vi "Main.vi"() -> ()   [LabVIEW 2014, in "LinksApplication.lvclass"]
uses:
  LinksApplication.lvclass
  Featherweight/Core/Actor/Instance/FTW-Actor.lvclass
  Featherweight/Core/Actor/Reference/FTW-ActorReference.lvclass
  Featherweight/Web/Server/FTW-WebService.lvclass
  <vilib>/wsapi/Web Request.lvclass
  Featherweight/Web/Utils/FTW-Web-HTTPResponseCode.ctl
  System.Windows.Forms
panel:
  in  "Canvas":refnum<k24>(container)
types:
  T1 = typedef "FTW-Web-HTTPResponseCode.ctl" = i32
  T2 = cluster{"Incoming HTTP Request":refnum<event-registration>}
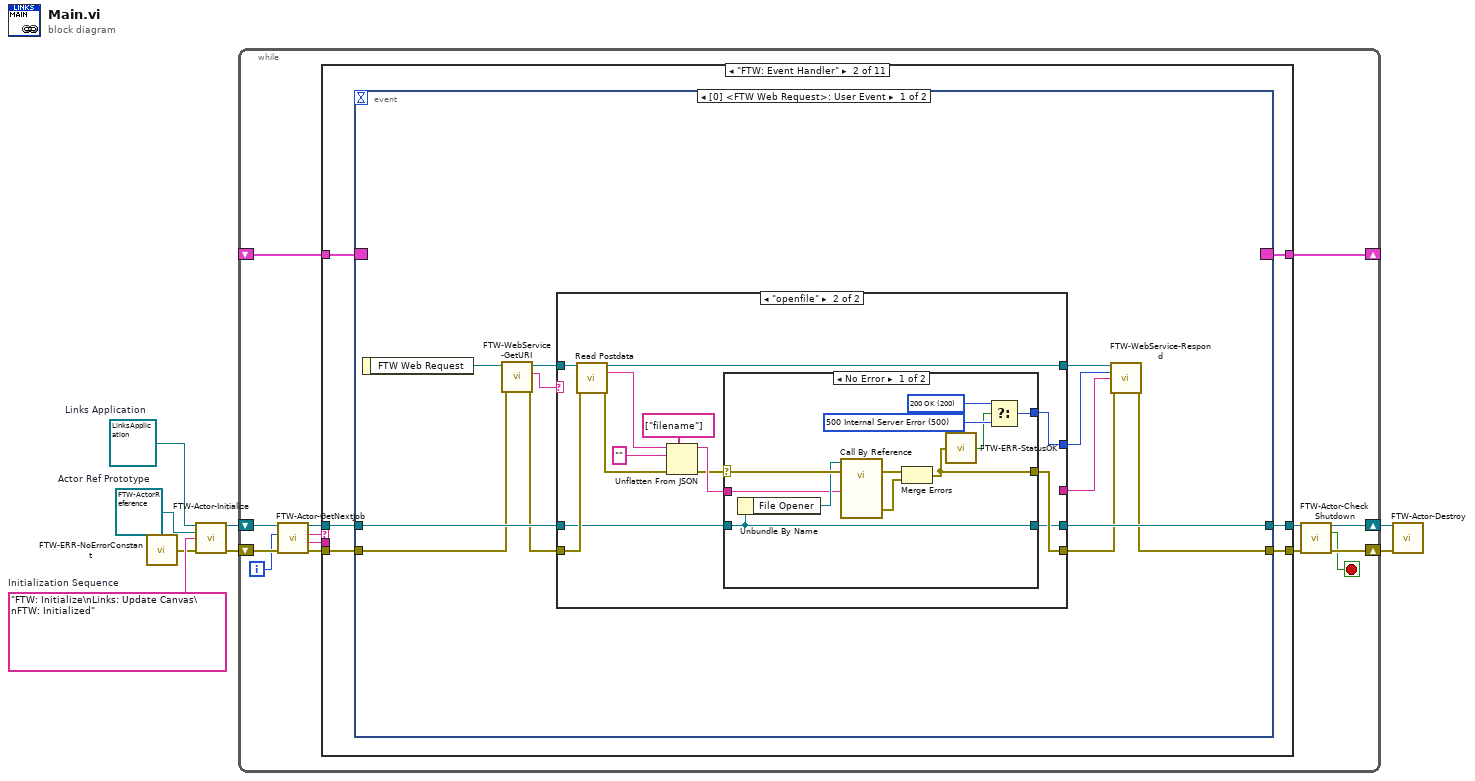
[diagram p0: block diagram]
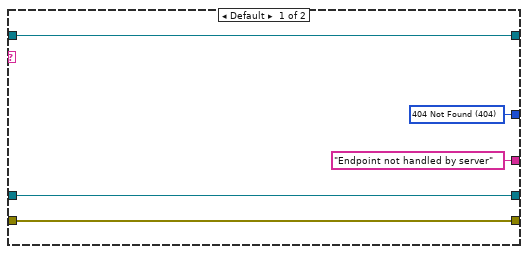
[diagram p3: hidden frame]
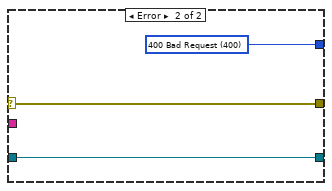
[diagram p4: hidden frame]
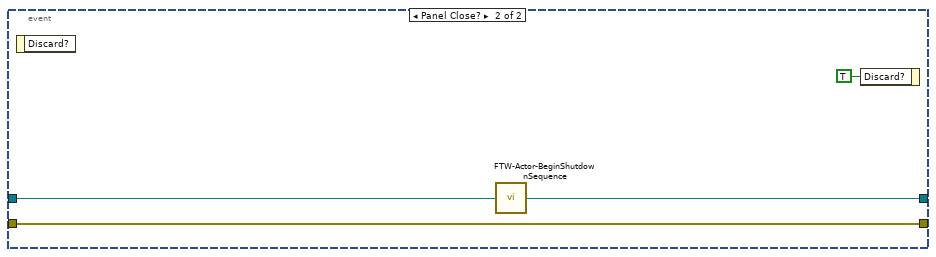
[diagram p5: hidden frame]
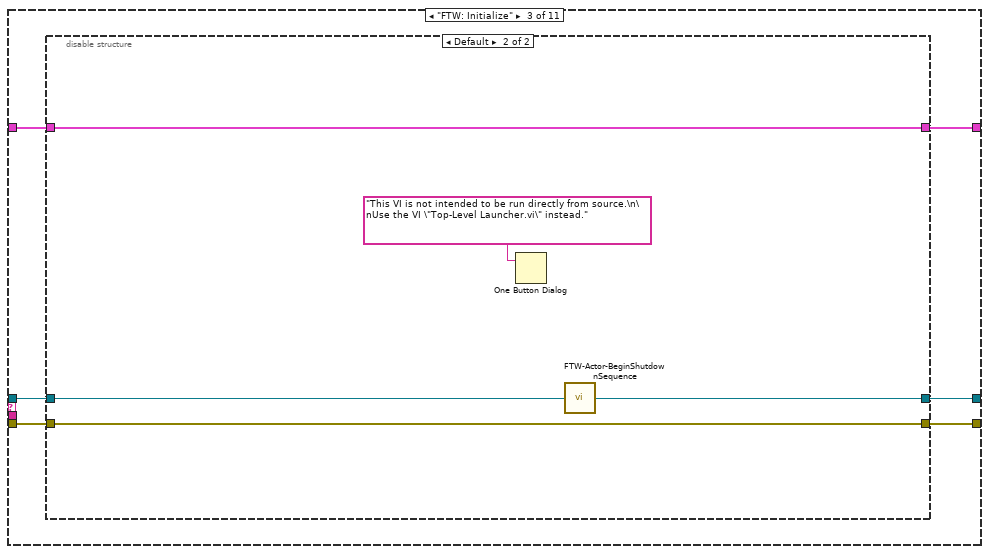
[diagram p6: hidden frame]
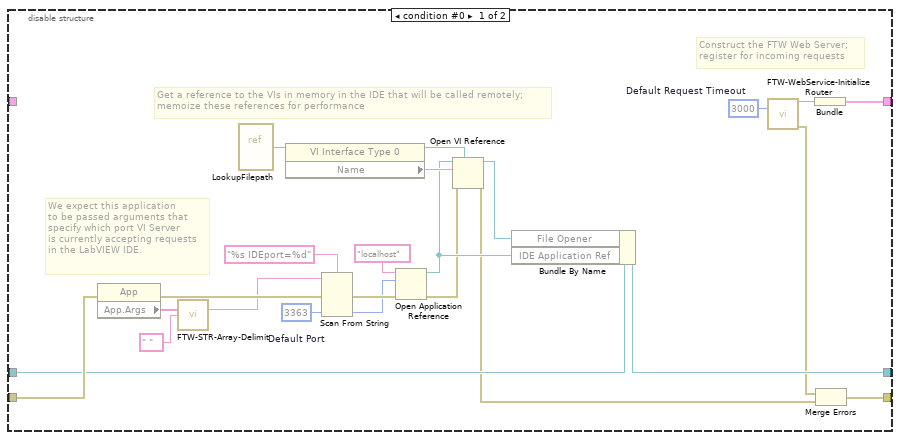
[diagram p7: hidden frame]
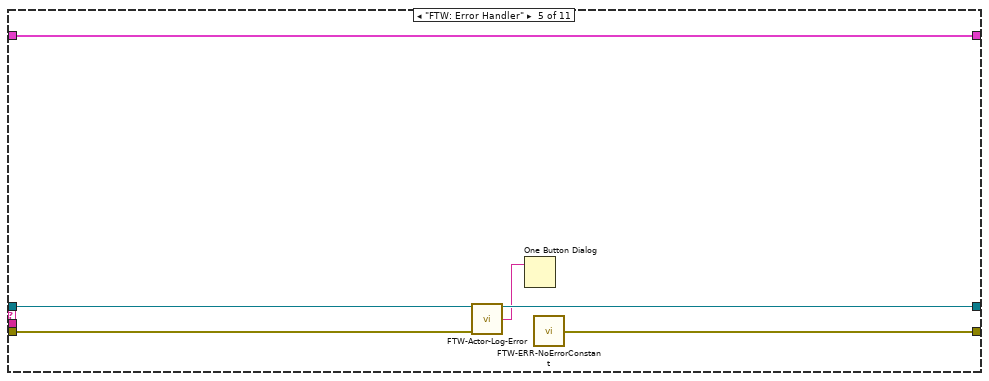
[diagram p9: hidden frame]
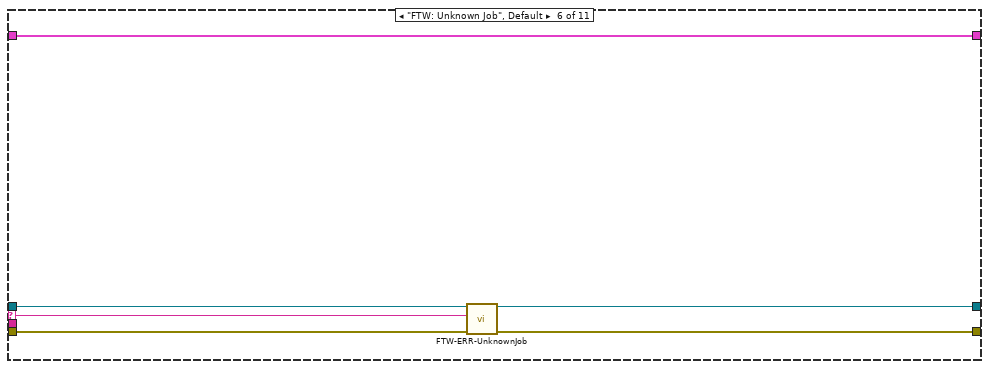
[diagram p10: hidden frame]
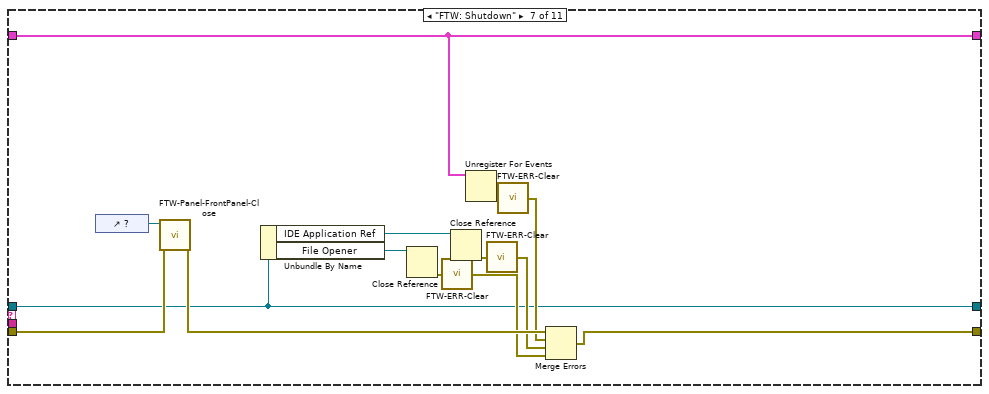
[diagram p11: hidden frame]
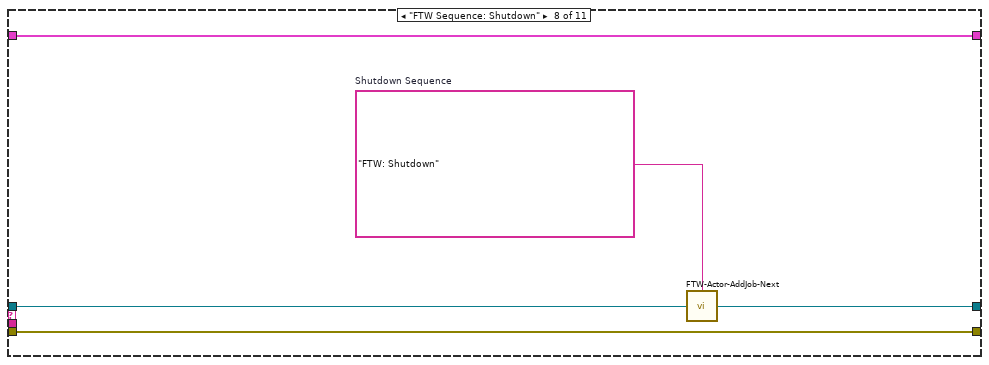
[diagram p12: hidden frame]
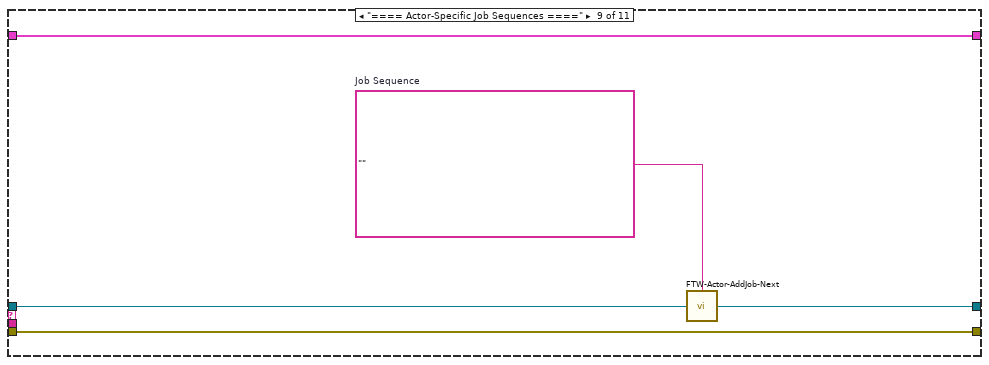
[diagram p13: hidden frame]
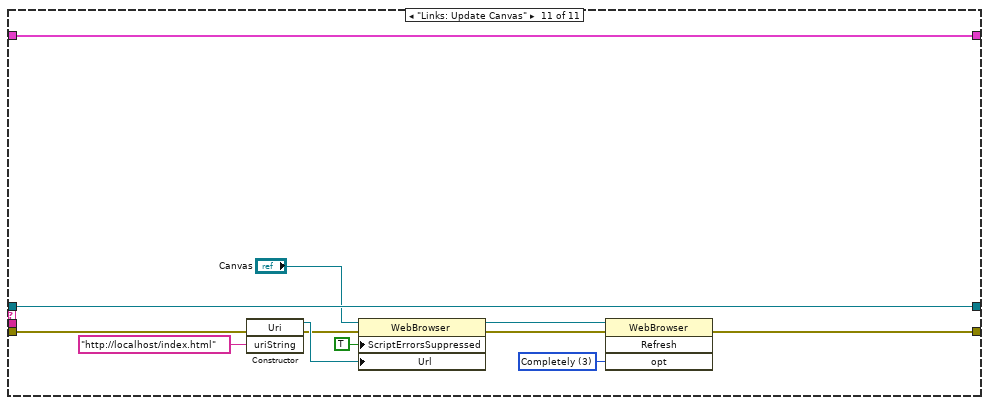
[diagram p15: hidden frame]
diagram:
  w1 = refnum<class "LinksApplication.lvclass"> refnum  # Links Application
  w3 = refnum<class "FTW-ActorReference.lvclass"> refnum  # Actor Ref Prototype
  w4 = "FTW: Initialize\nLinks: Update Canvas\nFTW: Initialized"  # Initialization Sequence
  n1 = call "FTW-ERR-NoErrorConstant.vi"() -> ("no error"=w2:errorcluster)
  n2 = call-dynamic "FTW-Actor-Initialize.vi"("Uninitialized FTW Actor"=w1, "Actor Ref Prototype"=w3, "Initialization Job Sequence"=w4, "error in"=w2) -> ("FTW Actor"=w8:refnum<class "LinksApplication.lvclass">, "error out"=w5:errorcluster)  [unwired: 10 in]
  n3 = while {
    shift-right: [w12] -> w6
    shift-left: w5 -> [w19]
    shift-right: [w9] -> _
    shift-left: _ -> [w22]
    shift-right: [w14] -> w7
    shift-left: w8 -> [w21]
    i -> [w10]
    stop <- w11 stop-if-true
    n4 = call "FTW-Actor-GetNextJob.vi"("error in"=w19, "Jobs Performed"=w10, "FTW Actor in"=w21) -> ("error out"=w18:errorcluster, "Job Data"=w16:string, "Job Name"=w17:string, "FTW Actor"=w20:refnum<class "LinksApplication.lvclass">)  [unwired: 5 in]
    n5 = case shown="\"FTW: Event Handler\"" w17 {
      selector: w17 -> [_ _ _ _ _ w124 _ _ _ _ _]
      tunnel: [w24 w31 w83 w117 w122 w125 w141 w146 w151 w155 w161] -> w13
      tunnel: w18 -> [w24 w30 w84 w117 w118 w126 w137 w146 w151 w155 w157]
      tunnel: w22 -> [w25 w28 w82 w116 w123 w128 w140 w147 w152 w154 w167]
      tunnel: [w25 w29 w85 w116 w123 w128 w140 w147 w152 w154 w167] -> w9
      tunnel: w16 -> [_ _ _ _ _ _ _ _ _ _ _]
      tunnel: [w23 w27 w81 w115 w120 w127 w129 w144 w149 w153 w166] -> w15
      tunnel: w20 -> [w23 w26 w80 w115 w121 w127 w129 w145 w150 w153 w166]
      frame "==== Featherweight Framework Jobs ====" {
      }
      frame "FTW: Event Handler" {
        n6 = event shown="[0] <FTW Web Request>: User Event" {
          selector: w28 -> [_ _]
          dyn-events: [_ _] -> w29
          timeout: _ -> [_ _]
          tunnel: [w34 w78] -> w31
          tunnel: w30 -> [w40 w78]
          tunnel: [w43 w76] -> w27
          tunnel: w26 -> [w42 w77]
          event User Event {
            n7 = event-data() -> ("FTW Web Request"=w41:refnum<class "FTW-WebService.lvclass">)  [unwired: 1 in]
            n8 = call "FTW-WebService-GetURI.vi"("error in"=w40, "FTW Web Request"=w41) -> ("error out"=w39:errorcluster, "RequestURI"=w32:string, "FTW Web Request out"=w38:refnum<class "FTW-WebService.lvclass">)  [unwired: 7 in]
            n9 = case shown="\"openfile\"" w32 {
              tunnel: [w46 w57] -> w33
              tunnel: w39 -> [w46 w60]
              tunnel: [w48 w49] -> w43
              tunnel: w42 -> [w48 w50]
              tunnel: w38 -> [w47 w61]
              tunnel: [w47 w58] -> w37
              tunnel: [w45 w59] -> w36
              tunnel: ["Endpoint not handled by server" ("Response Body") _] -> w35
              frame Default {
                w45 = T1 404 items=["100 Continue"=100, "101 Switching Protocols"=101, "200 OK"=200, "201 Created"=201, "202 Accepted"=202, "203 Non-Authoritative Information"=203, "204 No Content"=204, "205 Reset Content"=205, "206 Partial Content"=206, "300 Multiple Choices"=300, "301 Moved Permanently"=301, "302 Found"=302, "303 See Other"=303, "304 Not Modified"=304, "305 Use Proxy"=305, "306 (Unused)"=306, "307 Temporary Redirect"=307, "400 Bad Request"=400, "401 Unauthorized"=401, "402 Payment Required"=402, "403 Forbidden"=403, "404 Not Found"=404, "405 Method Not Allowed"=405, "406 Not Acceptable"=406, "407 Proxy Authentication Required"=407, "408 Request Timeout"=408, "409 Conflict"=409, "410 Gone"=410, "411 Length Required"=411, "412 Precondition Failed"=412, "413 Request Entity Too Large"=413, "414 Request-URI Too Long"=414, "415 Unsupported Media Type"=415, "416 Requested Range Not Satisfiable"=416, "417 Expectation Failed"=417, "500 Internal Server Error"=500, "501 Not Implemented"=501, "502 Bad Gateway"=502, "503 Service Unavailable"=503, "504 Gateway Timeout"=504, "505 HTTP Version Not Supported"=505] ("HTTP Response Code")
              }
              frame "openfile" {
                n10 = call <vilib>:"Read Postdata.vi"("LabVIEW Web Service Request"=w61, "error in (no error)"=w60) -> ("LabVIEW Web Service Request out"=w58:refnum<class "FTW-WebService.lvclass">, "postdata"=w53:string, "error out"=w54:errorcluster)  [unwired: 11 in]
                n11 = Unflatten From JSON(path=string[] ["filename"], JSON string=w53, type and defaults="", error in (no error)=w54) -> (value=w56:string, error out=w55:errorcluster)  [unwired: 3 in]
                n12 = case shown="No Error" w55 {
                  selector: w55 -> [w68 w75]
                  tunnel: [w70 w74] -> w59
                  tunnel: w56 -> [w62 _]
                  tunnel: [w64 w75] -> w57
                  tunnel: w50 -> [w63 w73]
                  tunnel: [w63 w73] -> w49
                  frame No Error {
                    w71 = T1 500 items=["100 Continue"=100, "101 Switching Protocols"=101, "200 OK"=200, "201 Created"=201, "202 Accepted"=202, "203 Non-Authoritative Information"=203, "204 No Content"=204, "205 Reset Content"=205, "206 Partial Content"=206, "300 Multiple Choices"=300, "301 Moved Permanently"=301, "302 Found"=302, "303 See Other"=303, "304 Not Modified"=304, "305 Use Proxy"=305, "306 (Unused)"=306, "307 Temporary Redirect"=307, "400 Bad Request"=400, "401 Unauthorized"=401, "402 Payment Required"=402, "403 Forbidden"=403, "404 Not Found"=404, "405 Method Not Allowed"=405, "406 Not Acceptable"=406, "407 Proxy Authentication Required"=407, "408 Request Timeout"=408, "409 Conflict"=409, "410 Gone"=410, "411 Length Required"=411, "412 Precondition Failed"=412, "413 Request Entity Too Large"=413, "414 Request-URI Too Long"=414, "415 Unsupported Media Type"=415, "416 Requested Range Not Satisfiable"=416, "417 Expectation Failed"=417, "500 Internal Server Error"=500, "501 Not Implemented"=501, "502 Bad Gateway"=502, "503 Service Unavailable"=503, "504 Gateway Timeout"=504, "505 HTTP Version Not Supported"=505] ("HTTP Response Code")
                    w72 = T1 200 items=["100 Continue"=100, "101 Switching Protocols"=101, "200 OK"=200, "201 Created"=201, "202 Accepted"=202, "203 Non-Authoritative Information"=203, "204 No Content"=204, "205 Reset Content"=205, "206 Partial Content"=206, "300 Multiple Choices"=300, "301 Moved Permanently"=301, "302 Found"=302, "303 See Other"=303, "304 Not Modified"=304, "305 Use Proxy"=305, "306 (Unused)"=306, "307 Temporary Redirect"=307, "400 Bad Request"=400, "401 Unauthorized"=401, "402 Payment Required"=402, "403 Forbidden"=403, "404 Not Found"=404, "405 Method Not Allowed"=405, "406 Not Acceptable"=406, "407 Proxy Authentication Required"=407, "408 Request Timeout"=408, "409 Conflict"=409, "410 Gone"=410, "411 Length Required"=411, "412 Precondition Failed"=412, "413 Request Entity Too Large"=413, "414 Request-URI Too Long"=414, "415 Unsupported Media Type"=415, "416 Requested Range Not Satisfiable"=416, "417 Expectation Failed"=417, "500 Internal Server Error"=500, "501 Not Implemented"=501, "502 Bad Gateway"=502, "503 Service Unavailable"=503, "504 Gateway Timeout"=504, "505 HTTP Version Not Supported"=505] ("HTTP Response Code")
                    n13 = Unbundle By Name(w63) -> ("File Opener"=w67:refnum<vi>)
                    n14 = call-by-ref "?"(reference=w67, error in=w68, "FileID"=w62) -> (error out=w66:errorcluster, 15:"error out"=w65:errorcluster)  [unwired: 14 in, 1 out]
                    n15 = Merge Errors(w66, w65) -> (w64:errorcluster)
                    n16 = call "FTW-ERR-StatusOK.vi"("error to check"=w64) -> ("Status OK?"=w69:bool)
                    n17 = Select(t=w72, s=w69, f=w71) -> (s? t:f=w70:T1)
                  }
                  frame Error {
                    w74 = T1 400 items=["100 Continue"=100, "101 Switching Protocols"=101, "200 OK"=200, "201 Created"=201, "202 Accepted"=202, "203 Non-Authoritative Information"=203, "204 No Content"=204, "205 Reset Content"=205, "206 Partial Content"=206, "300 Multiple Choices"=300, "301 Moved Permanently"=301, "302 Found"=302, "303 See Other"=303, "304 Not Modified"=304, "305 Use Proxy"=305, "306 (Unused)"=306, "307 Temporary Redirect"=307, "400 Bad Request"=400, "401 Unauthorized"=401, "402 Payment Required"=402, "403 Forbidden"=403, "404 Not Found"=404, "405 Method Not Allowed"=405, "406 Not Acceptable"=406, "407 Proxy Authentication Required"=407, "408 Request Timeout"=408, "409 Conflict"=409, "410 Gone"=410, "411 Length Required"=411, "412 Precondition Failed"=412, "413 Request Entity Too Large"=413, "414 Request-URI Too Long"=414, "415 Unsupported Media Type"=415, "416 Requested Range Not Satisfiable"=416, "417 Expectation Failed"=417, "500 Internal Server Error"=500, "501 Not Implemented"=501, "502 Bad Gateway"=502, "503 Service Unavailable"=503, "504 Gateway Timeout"=504, "505 HTTP Version Not Supported"=505] ("HTTP Response Code")
                  }
                }
              }
            }
            n18 = call "FTW-WebService-Respond.vi"("FTW Web Request"=w37, "HTTP Response Code"=w36, "Response Body"=w35, "error in"=w33) -> ("error out"=w34:errorcluster)  [unwired: 10 in, 1 out]
          }
          event Panel Close? {
            n19 = event-data() -> ()  [unwired: 1 in, 1 out]
            n20 = call "FTW-Actor-BeginShutdownSequence.vi"("FTW Actor"=w77) -> ("FTW Actor out"=w76:refnum<class "LinksApplication.lvclass">)  [unwired: 3 in]
            n21 = event-data("Discard?"=TRUE) -> ()  [unwired: 1 in, 1 out]
          }
        }
      }
      frame "FTW: Initialize" {
        n22 = disable-structure shown="Default" {
          disable-tunnel: [w109 w114] -> w85
          disable-tunnel: w84 -> [w106 w111]
          disable-tunnel: [w93 w111] -> w83
          disable-tunnel: w82 -> [_ w114]
          disable-tunnel: [w96 w112] -> w81
          disable-tunnel: w80 -> [w95 w113]
          frame condition #0 {
            w102 = u16 3363  # Default Port
            w107 = 3000  # Default Request Timeout
            # "We expect this application\nto be passed arguments that\nspecify which port VI Server\nis currently accepting requests\nin the LabVIEW IDE."
            # "Construct the FTW Web Server;\nregister for incoming requests"
            # "Get a reference to the VIs in memory in the IDE that will be called remotely;\nmemoize these references for performance"
            n23 = property class="App"(error in=w106) -> (error out=w104:errorcluster, "App.Args"=w105:string[])  [unwired: 1 in, 1 out]
            n24 = call "FTW-STR-Array-Delimit.vi"("Array of Strings"=w105, "Delimiter"=" ") -> ("Delimited String"=w100:string)  [unwired: 13 in]
            n25 = vi-ref "LookupFilepath.vi"() -> (w92:refnum<vi>)
            n26 = property class="VI Interface Type 0"(reference=w92) -> (reference out=w91:refnum<vi>, "Name"=w90:string)  [unwired: 1 in, 1 out]
            n27 = Scan From String(format string="%s IDEport=%d", input string=w100, error in=w104, default 2=w102) -> (error out=w101:errorcluster, output 2=w98:u16)  [unwired: 3 in, 2 out]
            n28 = Open Application Reference(8:w101, 10:w98, 11:"localhost" ("machine name (\"\":  open local reference)")) -> (0:w87:errorcluster, 3:w89:refnum<vi>)  [unwired: 1 in]
            n29 = Open VI Reference(type specifier VI Refnum (for type only)=w91, application reference (local)=w89, vi path=w90, error in (no error)=w87) -> (vi reference=w86:refnum<vi>, error out=w88:errorcluster)  [unwired: 2 in]
            n30 = Bundle By Name(cluster=w95, "File Opener"=w86, "IDE Application Ref"=w89) -> (w96:refnum<class "LinksApplication.lvclass">)
            n31 = call "FTW-WebService-InitializeRouter.vi"("Default Request Timeout"=w107) -> ("Incoming HTTP Request"=w108:refnum<event-registration>, "error out"=w94:errorcluster)  [unwired: 13 in]
            n32 = Bundle("Incoming HTTP Request"=w108) -> (w109:T2)  [unwired: 1 in]
            n33 = Merge Errors(w94, w88) -> (w93:errorcluster)
          }
          frame condition #1 (active) {
            n34 = One Button Dialog(message="This VI is not intended to be run directly from source.\n\nUse the VI \"Top-Level Launcher.vi\" instead.") -> ()  [unwired: 1 in, 1 out]
            n35 = call "FTW-Actor-BeginShutdownSequence.vi"("FTW Actor"=w113) -> ("FTW Actor out"=w112:refnum<class "LinksApplication.lvclass">)  [unwired: 3 in]
          }
        }
      }
      frame "FTW: Initialized" {
      }
      frame "FTW: Error Handler" {
        n36 = call-dynamic "FTW-Actor-Log-Error.vi"("Featherweight Actor"=w121, "Error to Log"=w118) -> ("Featherweight Actor out"=w120:refnum<class "LinksApplication.lvclass">, "Serialized Event"=w119:string)  [unwired: 11 in, 1 out]
        n37 = One Button Dialog(message=w119) -> ()  [unwired: 1 in, 1 out]
        n38 = call "FTW-ERR-NoErrorConstant.vi"() -> ("no error"=w122:errorcluster)
      }
      frame "FTW: Unknown Job", Default {
        n39 = call "FTW-ERR-UnknownJob.vi"("error in"=w126, "Unknown Job"=w124) -> ("error out"=w125:errorcluster)  [unwired: 9 in]
      }
      frame "FTW: Shutdown" {
        n40 = control-ref of="?"() -> (w136:refnum<vi>)
        n41 = call "FTW-Panel-FrontPanel-Close.vi"("error in"=w137, "VI Ref"=w136) -> ("error out"=w142:errorcluster)  [unwired: 8 in, 1 out]
        n42 = Unbundle By Name(w129) -> ("IDE Application Ref"=w135:refnum<vi>, "File Opener"=w134:refnum<vi>)
        n43 = Close Reference(reference=w134) -> (error out=w133:errorcluster)  [unwired: 1 in]
        n44 = call "FTW-ERR-Clear.vi"("error to snuff"=w133) -> ("no error"=w130:errorcluster)
        n45 = Close Reference(reference=w135) -> (error out=w132:errorcluster)  [unwired: 1 in]
        n46 = Unregister For Events(event registration refnum=w140) -> (error out=w139:errorcluster)  [unwired: 1 in]
        n47 = call "FTW-ERR-Clear.vi"("error to snuff"=w132) -> ("no error"=w131:errorcluster)
        n48 = call "FTW-ERR-Clear.vi"("error to snuff"=w139) -> ("no error"=w138:errorcluster)
        n49 = Merge Errors(w142, w138, w131, w130) -> (w141:errorcluster)
      }
      frame "FTW Sequence: Shutdown" {
        w143 = "FTW: Shutdown"  # Shutdown Sequence
        n50 = call "FTW-Actor-AddJob-Next.vi"("Add Next in Job Queue"=w143, "FTW Actor"=w145) -> ("FTW Actor out"=w144:refnum<class "LinksApplication.lvclass">)  [unwired: 2 in]
      }
      frame "==== Actor-Specific Job Sequences ====" {
        w148 = ""  # Job Sequence
        n51 = call "FTW-Actor-AddJob-Next.vi"("Add Next in Job Queue"=w148, "FTW Actor"=w150) -> ("FTW Actor out"=w149:refnum<class "LinksApplication.lvclass">)  [unwired: 2 in]
      }
      frame "==== Actor-Specific Jobs ====" {
      }
      frame "Links: Update Canvas" {
        w159 = 3 items=["Normal", "IfExpired", "Continue", "Completely"] ("opt")
        n52 = constructor class="Uri"(error in=w157, "uriString"="http://localhost/index.html" ("urlString")) -> (reference out=w160:refnum<k24>, error out=w156:errorcluster)  [unwired: 2 in, 2 out]
        n53 = property class="WebBrowser"(reference="Canvas", error in=w156, "ScriptErrorsSuppressed"=TRUE, "Url"=w160) -> (reference out=w162:refnum<k24>, error out=w163:errorcluster)
        n54 = invoke class="WebBrowser" method="Refresh"(reference=w162, error in=w163, "opt"=w159) -> (error out=w161:errorcluster)  [unwired: 1 in, 3 out]
      }
    }
    n55 = call "FTW-Actor-CheckShutdown.vi"("FTW Actor in"=w15, "error in"=w13) -> ("FTW Actor"=w14:refnum<class "LinksApplication.lvclass">, "Shutdown?"=w11:bool, "error out"=w12:errorcluster)  [unwired: 11 in]
  }
  n56 = call-dynamic "FTW-Actor-Destroy.vi"("FTW Actor"=w7, "error in"=w6) -> ()  [unwired: 13 in, 1 out]
